vi "main_80MHz.vi"() -> ()   [LabVIEW 2010]
uses:
  common_typedefs/channels_cluster.ctl
  common_typedefs/gate_parameters_cluster.ctl
  common_typedefs/pixel_to_host_enum.ctl
  <vilib>/Platform/TimedLoop/XDataNode/XDataNode.xnode
  <vilib>/Platform/TimedLoop/XDataNode/timing_clust.ctl
  <vilib>/Platform/TimedLoop/XDataNode/nitl_modes.ctl
  <vilib>/Platform/TimedLoop/XDataNode/wakeup.ctl
  <vilib>/eio/EIONode/EIONode.xnode
  <vilib>/rvi/eio/nirviEIOImplementation/nirviEIOImplementation.xnode
  <vilib>/rvi/eio/common/nirviEmuClasses.ctl
  <vilib>/rvi/eio/common/nirviEmuTemplateMethod_noerrors.vi
  <vilib>/Platform/TimedLoop/XDataNode/XDNodeRunTimeDep.lvlib
  common_VIs/OnBoardBuffer/OnBoardBuffer.lvlib
panel:
  in  "pixel-to-host mode":T1
  in  "gate 3":T2
  in  "gate 2":T2
  in  "gate 1":T2
  out "integrated pixel values":T3
  out "data read":T3
  in  "channel offsets":T3
  out "clock 3 state":bool
  out "clock 2 state":bool
  out "clock 1 state":bool
  in  "stop acquisition at FIFO overflow?":bool=TRUE
  in  "wait for trigger?":bool
  in  "stop":bool
  in  "acquire":bool
  out "acquiring?":bool
  out "FIFO overflow":bool
  out "current pixel no.":i64
  in  "number of pixels":i64=-1
  in  "maximum bit depth":i8
  in  "iterations per pixel":u32
  in  "enable ADC clock?":bool=TRUE
  in  "ADC clock phase":u8
  in  "converter box version":i16=1 min=1 max=2
  # "Outputs / displays"
  # "Integration parameters"
  # "Clock parameters"
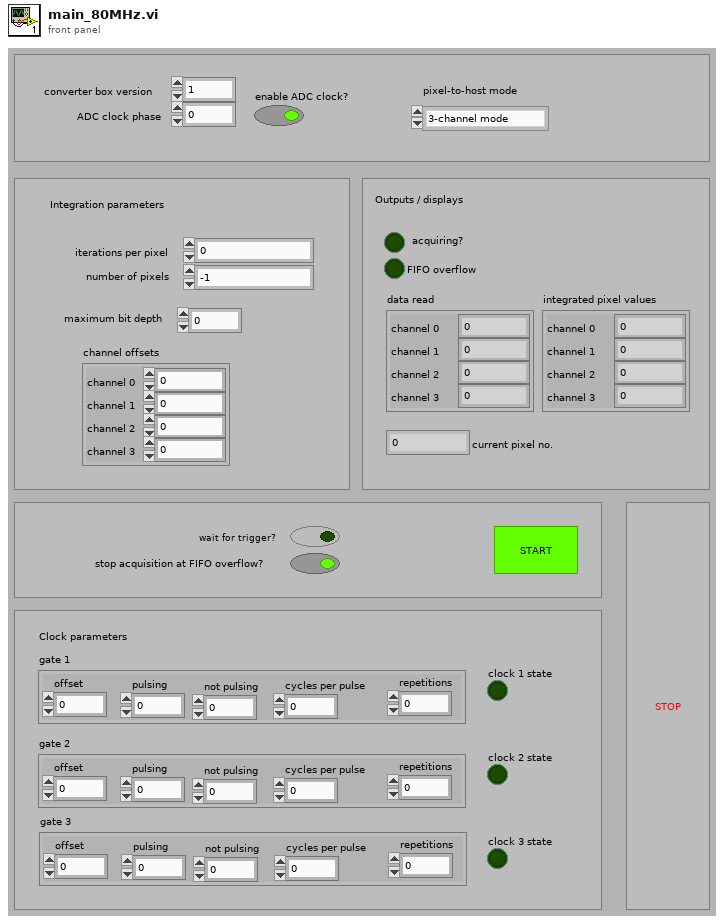
[diagram p1: front panel]
types:
  T1 = typedef "pixel_to_host_enum.ctl" = enum16{"3-channel mode", "4-channel mode"}
  T2 = typedef "gate_parameters_cluster.ctl" = cluster{"offset":i64, "pulsing":i64, "not pulsing":i64, "cycles per pulse":i64, "repetitions":i64}
  T3 = typedef "channels_cluster.ctl" = cluster{"channel 0":u32, "channel 1":u32, "channel 2":u32, "channel 3":u32}
  T4 = typedef "OnBoardBuffer.lvlib/buffer_state_cluster.ctl" = cluster{"depth":u32, "current read address":u32, "current write address":u32}
  T5 = typedef "XDNodeRunTimeDep.lvlib/timing_clust.ctl" = cluster{"Expected End [f-1]":u64, "Actual End [f-1]":u64, "Finished Late? [f-1]":bool, "Expected End [i-1]":u64, "Actual End [i-1]":u64, "Finished Late? [i-1]":bool, "Expected Start [i]":u64, "Actual Start [i]":u64, "Expected Start [f]":u64, "Actual Start [f]":u64, "Source Name":string, "Structure Name":string, "Period":i64, "Deadline":i64, "Offset":i64, "Start":i64, "Priority":i32, "Timeout":i32, "Mode":T6, "Wakeup Reason":T7, "Error":errorcluster, "Source Type":string, "Secondary Source Type":string, "Global End Time":u64, "Global Start Time":u64, "Frame Duration":u64, "Iteration Duration":u64, "Assigned CPU":i32, "I/O Scan Engine Mode":u32}
  T6 = typedef "XDNodeRunTimeDep.lvlib/nitl_modes.ctl" = enum32{"No Change", "Process missed periods, maintain original phase", "Discard missed periods, maintain original phase", "Process missed periods, ignore original phase", "Discard missed periods, ignore original phase"}
  T7 = typedef "XDNodeRunTimeDep.lvlib/wakeup.ctl" = enum32{"Normal", "Aborted", "Asynchronous wakeup", "Timing source error", "Timed loop error", "Timeout"}
  T8 = typedef "buffers_state_array.ctl" = T4[]
  T9 = typedef "nirviEmuClasses.ctl" = enum16{"IO Read", "IO Write", "Method", "Property Read", "Property Write"}
  T10 = typedef "gate_counters_cluster.ctl" = cluster{"phase iteration counter":i64, "phase repetition counter":i64, "pulse iteration counter":i64, "phase state":bool}
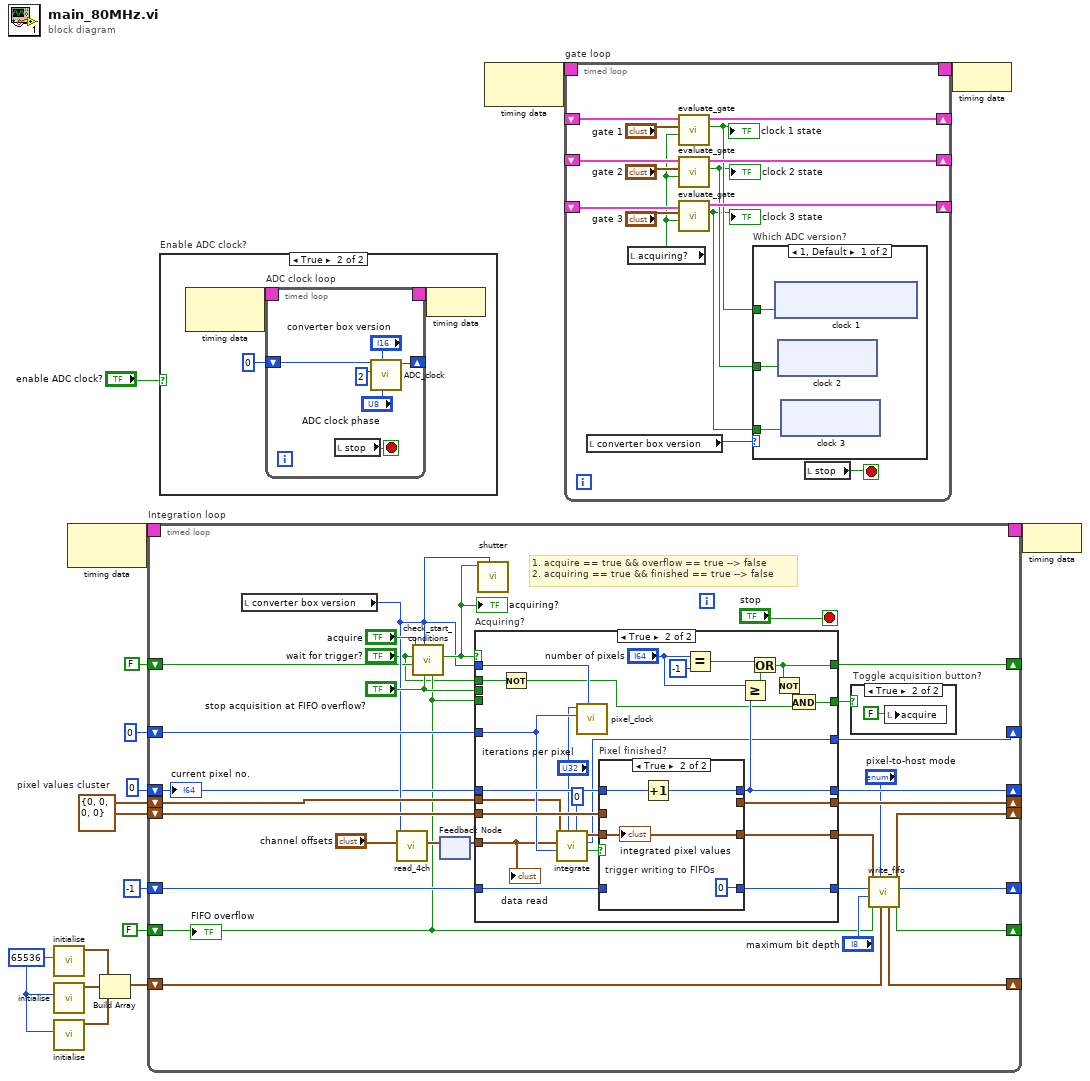
[diagram p0: block diagram]
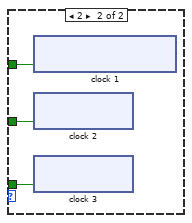
[diagram p2: hidden frame]
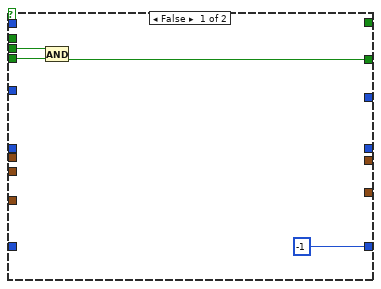
[diagram p4: hidden frame]
diagram:
  w5 = u32 65536 ("depth")
  w9 = T3 {"channel 0"=0, "channel 1"=0, "channel 2"=0, "channel 3"=0}  # pixel values cluster
  n1 = call "initialise.vi"("depth"=w5) -> ("buffer state"=w2:T4)  [unwired: 10 in]
  n2 = call "initialise.vi"("depth"=w5) -> ("buffer state"=w3:T4)  [unwired: 10 in]
  n3 = call "initialise.vi"("depth"=w5) -> ("buffer state"=w4:T4)  [unwired: 10 in]
  n4 = node-c288() -> (w15:T5)  [unwired: 1 in]
  n5 = Build Array(w2, w3, w4) -> (w1:T4[])
  n6 = timed-loop "Integration loop" {
    timing: w15 -> [_]
    timing-out: [_] -> w14
    shift-right: [w39] -> _
    shift-left: i64 0 -> [w24]
    shift-right: [w38] -> _
    shift-left: u32 0 ("iteration counter out") -> [w42]
    shift-right: [w40] -> _
    shift-left: w9 -> [w44]
    shift-right: [w25] -> _
    shift-left: FALSE -> [w21]
    shift-right: [w30] -> _
    shift-left: w9 -> [w41]
    shift-right: [w27] -> _
    shift-left: -1 ("block index out") -> [w43]
    shift-right: [w33] -> _
    shift-left: FALSE -> [w22]
    shift-right: [w18] -> _
    shift-left: w1 -> [w17]
    stop <- "stop" stop-if-true
    # "1. acquire == true && overflow == true --> false\n2. acquiring == true && finished == true --> false"
    n7 = local read "converter box version"() -> (w31:i16)
    n8 = call "read_4ch.vi"("channel offsets"="channel offsets", "converter box version"=w31) -> ("read output"=w36:T3)  [unwired: 9 in]
    n9 = call "check_start_conditions.vi"("FIFO overflow?"=w21, "stop at FIFO overflow?"="stop acquisition at FIFO overflow?", "converter box version"=w31, "already acquiring?"=w22, "in triggered mode?"="wait for trigger?", "acquire"="acquire") -> ("acquire?"=w32:bool)  [unwired: 5 in]
    "acquiring?" <- w32
    n10 = feedback-in #1(w36) -> ()
    n11 = feedback #1() -> (w35:T3)  [unwired: 1 in]
    n12 = case "Acquiring?" shown="True" w32 {
      tunnel: w31 -> [_ w76]
      tunnel: [_ w58] -> w29
      tunnel: [_ w66] -> w38
      tunnel: [_ w72] -> w39
      tunnel: w44 -> [_ w63]
      tunnel: w43 -> [_ w61]
      tunnel: w24 -> [_ w70]
      tunnel: w42 -> [_ w65]
      tunnel: w41 -> [_ w69]
      tunnel: [_ w71] -> w40
      tunnel: [-1 ("block index out") w59] -> w26
      tunnel: w35 -> [_ w64]
      tunnel: "stop acquisition at FIFO overflow?" -> [w50 _]
      tunnel: [_ w56] -> w33
      tunnel: [w48 w53] -> w19
      tunnel: w21 -> [w49 _]
      tunnel: "wait for trigger?" -> [_ w55]
      frame False {
        n13 = And(x=w49, y=w50) -> (x .and. y?=w48:bool)
      }
      frame True {
        n14 = Not(x=w55) -> (.not. x?=w52:bool)
        n15 = call "integrate.vi"("waiting iterations per pixel"=u32 0, "integration iterations per pixel"="iterations per pixel", "iteration counter in"=w65, "sampling values in"=w64, "previous pixel values in"=w63) -> ("finished?"=w68:bool, "iteration counter out"=w66:u32, "new pixel values out"=w67:T3)  [unwired: 4 in]
        n16 = call "pixel_clock.vi"("converter box version"=w76, "current iteration"=w65, "iterations per pixel"="iterations per pixel") -> ()  [unwired: 9 in]
        n17 = case "Pixel finished?" shown="True" w68 {
          tunnel: w67 -> [w80 w84]
          tunnel: [w79 w84] -> w58
          tunnel: [w78 w82] -> w72
          tunnel: w70 -> [w78 w83]
          tunnel: [w80 _] -> w71
          tunnel: w69 -> [w79 _]
          tunnel: w61 -> [w77 _]
          tunnel: [w77 w81] -> w59
          frame False {
          }
          frame True {
            w81 = 0  # trigger writing to FIFOs
            n18 = Increment(x=w83) -> (x+1=w82:i64)
            "integrated pixel values" <- w84
          }
        }
        n19 = Equal?(x="number of pixels", y=i64 -1 ("x")) -> (x = y?=w75:bool)
        n20 = Greater Or Equal?(x="number of pixels", y=w72) -> (x >= y?=w74:bool)
        n21 = Or(x=w75, y=w74) -> (x .or. y?=w56:bool)
        n22 = Not(x=w56) -> (.not. x?=w54:bool)
        n23 = And(x=w54, y=w52) -> (x .and. y?=w53:bool)
        "data read" <- w64
      }
    }
    n24 = call "shutter.vi"("converter box version"=w31, "open?"=w32) -> ()  [unwired: 10 in]
    n25 = case "Toggle acquisition button?" shown="True" w19 {
      frame False {
      }
      frame True {
        n26 = local write "acquire"(FALSE) -> ()
      }
    }
    n27 = call "write_fifo.vi"("buffers state in"=w17, "pixel-to-host\n mode"="pixel-to-host mode", "FIFO overflow in"=w21, "maximum bit depth"="maximum bit depth", "block index in"=w26, "values to be written"=w29) -> ("FIFO overflow out"=w25:bool, "block index out"=w27:i32, "channels out"=w30:T3, "buffers state out"=w18:T8)  [unwired: 2 in]
    "current pixel no." <- w24
    "FIFO overflow" <- w21
  }
  n28 = case "Enable ADC clock?" shown="True" "enable ADC clock?" {
    frame False {
    }
    frame True {
      n29 = node-c288() -> (w89:T5)  [unwired: 1 in]
      n30 = timed-loop "ADC clock loop" {
        timing: w89 -> [_]
        timing-out: [_] -> w88
        shift-right: [w94] -> _
        shift-left: u8 0 ("counter out") -> [w95]
        stop <- w91 stop-if-true
        n31 = local read "stop"() -> (w91:bool)
        n32 = call "ADC_clock.vi"("phase"="ADC clock phase", "converter box version"="converter box version", "iterations per cycle"=u8 2, "counter in"=w95) -> ("counter out"=w94:u8)  [unwired: 7 in]
      }
      n33 = node-c288(w88) -> ()
    }
  }
  n34 = node-c288() -> (w8:T5)  [unwired: 1 in]
  n35 = timed-loop "gate loop" {
    timing: w8 -> [_]
    timing-out: [_] -> w7
    shift-right: [w113] -> _
    shift-left: _ -> [w114]
    shift-right: [w111] -> _
    shift-left: _ -> [w112]
    shift-right: [w110] -> _
    shift-left: _ -> [w109]
    stop <- w104 stop-if-true
    n36 = local read "converter box version"() -> (w103:i16)
    n37 = local read "acquiring?"() -> (w105:bool)
    n38 = call "evaluate_gate.vi"("acquiring?"=w105, "gate settings"="gate 1", "gate counters in"=w114) -> ("pulse state out"=w102:bool, "gate counters out"=w113:T10)  [unwired: 7 in]
    "clock 1 state" <- w102
    n39 = call "evaluate_gate.vi"("acquiring?"=w105, "gate settings"="gate 2", "gate counters in"=w112) -> ("pulse state out"=w101:bool, "gate counters out"=w111:T10)  [unwired: 7 in]
    "clock 2 state" <- w101
    n40 = call "evaluate_gate.vi"("acquiring?"=w105, "gate settings"="gate 3", "gate counters in"=w109) -> ("pulse state out"=w100:bool, "gate counters out"=w110:T10)  [unwired: 7 in]
    "clock 3 state" <- w100
    n41 = case "Which ADC version?" shown="1, Default" w103 {
      tunnel: w102 -> [w115 w153]
      tunnel: w101 -> [w116 w152]
      tunnel: w100 -> [w117 w151]
      frame 1, Default {
        n42 = xnode "clock 1"("Connector1/DIO32"=w115) -> ()  [unwired: 1 in, 1 out]
        n43 = xnode "clock 2"("PXI_RTSI_1"=w116) -> ()  [unwired: 1 in, 1 out]
        n44 = xnode "clock 3"("PXI_RTSI_2"=w117) -> ()  [unwired: 1 in, 1 out]
      }
      frame 2 {
        n45 = xnode "clock 1"("Connector0/DIO38"=w153) -> ()  [unwired: 1 in, 1 out]
        n46 = xnode "clock 2"("PXI_RTSI_1"=w152) -> ()  [unwired: 1 in, 1 out]
        n47 = xnode "clock 3"("PXI_RTSI_2"=w151) -> ()  [unwired: 1 in, 1 out]
      }
    }
    n48 = local read "stop"() -> (w104:bool)
  }
  n49 = node-c288(w7) -> ()
  n50 = node-c288(w14) -> ()
